vi "Pre Launch Init.vi"(11 "Network Stream Writer in":refnum<class "Network Stream Writer.lvclass">) -> (0 "error out":errorcluster, 3 "Network Stream Writer out":refnum<class "Network Stream Writer.lvclass">)   [LabVIEW 2014, in "Network Stream Writer.lvlib" / "Network Stream Writer.lvclass"]
doc: "(<B>Filename</B>: Actor Framework.lvlib:Actor.lvclass:Pre Launch Init.vi)\n\nDefines behavior that occurs after the Launch Nested Actor method is invoked but before the actor's Actor Core method begins running.\n\nBy default, this method does nothing. A descendant class may override it to define behavior."
uses:
  Network Stream Writer.lvclass
  Network Stream/Network Stream/Network Stream.lvclass
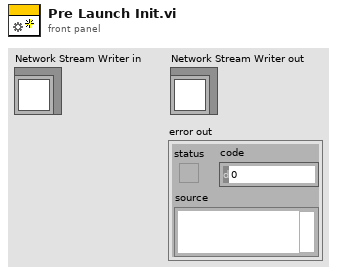
[diagram p1: front panel]
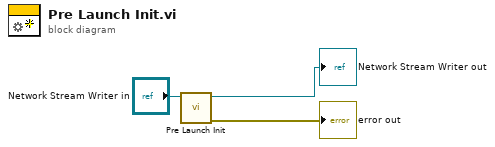
[diagram p0: block diagram]
diagram:
  n1 = call-parent "Pre Launch Init.vi"("Actor in"="Network Stream Writer in") -> ("error out"=→"error out":errorcluster, "Actor out"=→"Network Stream Writer out":refnum<class "Network Stream Writer.lvclass">)  [unwired: 9 in]
